vi "_Read16Instruction.vi"(6 "error in (no error)":errorcluster, 8 "Address In":i16, 9 "Refnum in":refnum<k21>) -> (0 "error out":errorcluster, 1 "Value":i16, 2 "Address Out":i16, 3 "Refnum Out":refnum<k21>)   [LabVIEW 2018, in "Modbus_Processing_Unit.lvlib" / "MPU.lvclass"]
uses:
  MPU.lvclass
  <vilib>/rvi/DataTransferAndStorage/Container/Common/niFpgaContainerExecOnDevCompGetState.vi
  <vilib>/rvi/Emulation/niFpgaEmulationIsFPGAContextNoSignature.vi
  <vilib>/rvi/DataTransferAndStorage/Container/Common/niFpgaContainerGetUniqueNameForEmu.vi
  <vilib>/rvi/Emulation/niFpgaProcessEmulError.vi
  <vilib>/rvi/Emulation/niFpgaSctlEmulationGetInTimedLoop.vi
  <vilib>/rvi/errors/nirviReportUnexpectedCaseInternalError (U32).vi
  <vilib>/rvi/Memory/Memory_Emulation/niFpgaMemoryEmulationCacheClearOnFirstRun.vi
  <vilib>/rvi/Memory/Memory_Emulation/nirvimemoryEmulationManagerCache_MakeExclusive.vi
  <vilib>/rvi/Memory/Memory_Emulation/niFpgaMemoryEmulationValidateCache.vi
  <vilib>/rvi/Memory/Memory_Emulation/nirvimemoryEmulationManagerCache_InsertValue.vi
  <vilib>/Utility/error.llb/Clear Errors.vi
  <vilib>/rvi/Memory/Memory_Emulation/nirvimemoryEmulationManagerCache_ReleaseExclusive.vi
  <vilib>/rvi/Memory/Memory_Emulation/nirvimemoryEmulationManagerCache_GetValue.vi
  <vilib>/rvi/Memory/Memory_Emulation/nirvimemoryEmulationManagerCache_SetValue.vi
  <vilib>/rvi/Emulation/niFpgaSctlEmulationResourceMgr.vi
  <vilib>/rvi/DataTransferAndStorage/Container/XNode/niFpgaContainer.xnode
  <vilib>/rvi/Memory/Memory_Emulation/niFpgaMemoryEmulationRefIn.vi
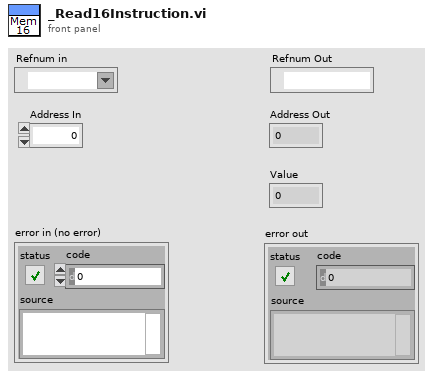
[diagram p1: front panel]
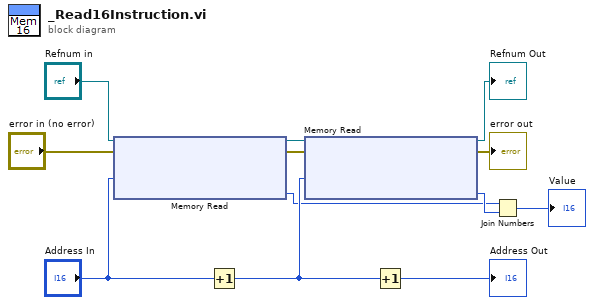
[diagram p0: block diagram]
diagram:
  n1 = xnode "Memory Read"("Address"="Address In", "error in (no error)"="error in (no error)", "Memory In"="Refnum in") -> ("Data"=w8:u8, "error out"=w10:errorcluster, "Memory Out"=w9:refnum<k21>)
  n2 = Increment(x="Address In") -> (x+1=w11:i16)
  n3 = xnode "Memory Read"("Address"=w11, "error in (no error)"=w10, "Memory In"=w9) -> ("Data"=w12:u8, "error out"=→"error out":errorcluster, "Memory Out"=→"Refnum Out":refnum<k21>)
  n4 = Increment(x=w11) -> (x+1=→"Address Out":i16)
  n5 = Join Numbers(hi=w8, lo=w12) -> ((hi.lo)=→"Value":u16)
